vi "Get Tables.vi"(8 "error in (no error)":errorcluster, 11 "DBMS in":refnum<class "DBMS.lvclass">) -> (0 "error out":errorcluster, 2 "Table Array":string[](array[string]), 3 "DBMS out":refnum<class "DBMS.lvclass">, 10 "System Tables (false)":bool)   [LabVIEW 2020, in "DBMS.lvclass"]
uses:
  DBMS.lvclass
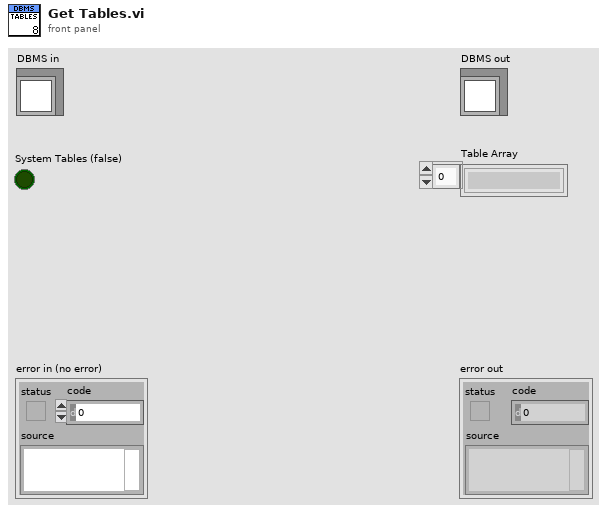
[diagram p1: front panel]
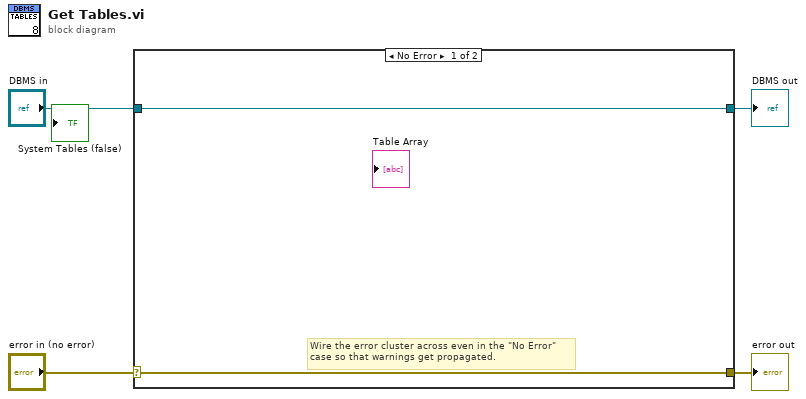
[diagram p0: block diagram]
diagram:
  n1 = case shown="No Error" "error in (no error)" {
    selector: "error in (no error)" -> [w5 w8]
    tunnel: [w5 w8] -> w3
    tunnel: [w6 w7] -> w1
    tunnel: "DBMS in" -> [w6 w7]
    frame No Error {
      # "Wire the error cluster across even in the \"No Error\"\ncase so that warnings get propagated."
    }
    frame Error {
    }
  }
  "error out" <- w3
  "DBMS out" <- w1
